vi "Workspace.UI.Pull.vi"(8 "error in (no error)":errorcluster, 11 "UI.Refs":T1) -> (0 "error out":errorcluster, 2 "Value":dbl)   [LabVIEW 2019, in "Diagnostics Workspace Shared.lvlib"]
uses:
  Shared/Types/UI.Refs.ctl
  Shared/Types/Command.New.ctl
  Diagnostics Workspace Shared.lvlib
  Shared/Diagnostics Addon Shared.lvlib
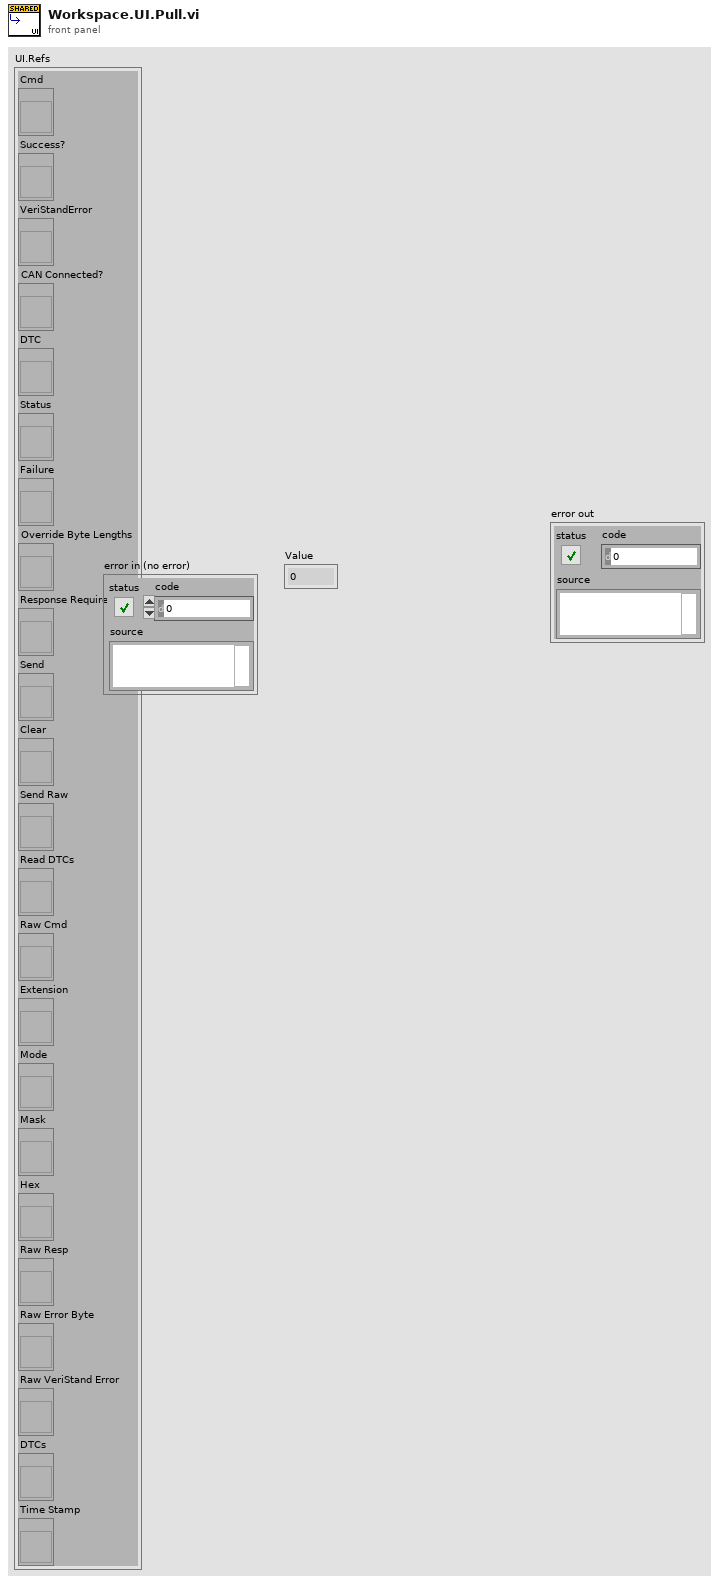
[diagram p1: front panel]
types:
  T1 = typedef "Diagnostics Addon Shared.lvlib/UI.Refs.ctl" = cluster{"Cmd":refnum<vi>, "Success?":refnum<vi>, "VeriStandError":refnum<vi>, "CAN Connected?":refnum<vi>, "DTC":refnum<vi>, "Status":refnum<vi>, "Failure":refnum<vi>, "Override Byte Lengths":refnum<vi>, "Response Required?":refnum<vi>, "Send":refnum<vi>, "Clear":refnum<vi>, "Send Raw":refnum<vi>, "Read DTCs":refnum<vi>, "Raw Cmd":refnum<vi>, "Extension":refnum<vi>, "Mode":refnum<vi>, "Mask":refnum<vi>, "Hex":refnum<vi>, "Raw Resp":refnum<vi>, "Raw Error Byte":refnum<vi>, "Raw VeriStand Error":refnum<vi>, "DTCs":refnum<vi>, "Time Stamp":refnum<vi>}
  T2 = typedef "Command.New.ctl" = enum8{"None", "Clear Status Channels", "Read All DIDs", "Read All PIDs", "Configure and Start DPIDs", "Stop DPIDs"}
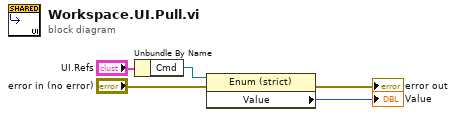
[diagram p0: block diagram]
diagram:
  n1 = Unbundle By Name("UI.Refs") -> ("Cmd"=w4:refnum<vi>)
  n2 = property class="Enum (strict)"(reference=w4, error in="error in (no error)") -> (error out=→"error out":errorcluster, "Value"=→"Value":T2)  [unwired: 1 out]
